vi "Save-Recall Instrument Settings.vi"(8 "error in (no error)":errorcluster, 9 "Memory Location (1)":i32(ring)=1 items=["1"=1, "2"=2, "3"=3, "4"=4], 10 "Operation (0: Save)":u16(ring) items=["Save", "Recall"], 11 "VISA resource name":refnum<visa-resource-name>) -> (0 "error out":errorcluster, 3 "VISA resource name out":refnum<visa-resource-name>)   [LabVIEW 2020, in "Agilent 34401.lvlib"]
doc: "Allows users to save or recall instrument mode at a specific memory location.\n\n<B>Note:</B>\n\n(1) This VI only applies to the 34410/34411 models.\n\n(2) Low-level <B>Initiate Measurement</B> and <B>Fetch Measurement</B> VIs must be used to transfer data from the instrument after a Recall operation. Higher level VIs like Read, configure instrument parameters that can differ from those recalled with this VI."
uses:
  Agilent 34401.lvlib
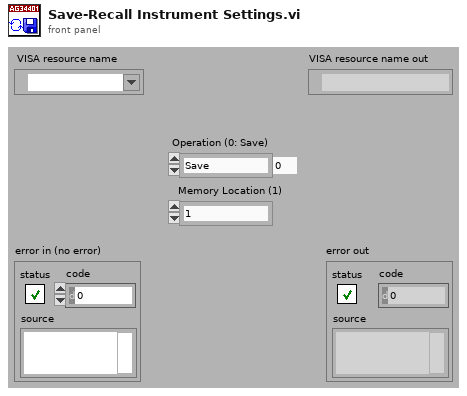
[diagram p1: front panel]
types:
  T1 = typedef "Agilent 34401.lvlib/Extended User Data.ctl" = cluster{"Trigger Source":u16, "Math Storage":u16, "Agilent Model":i32}
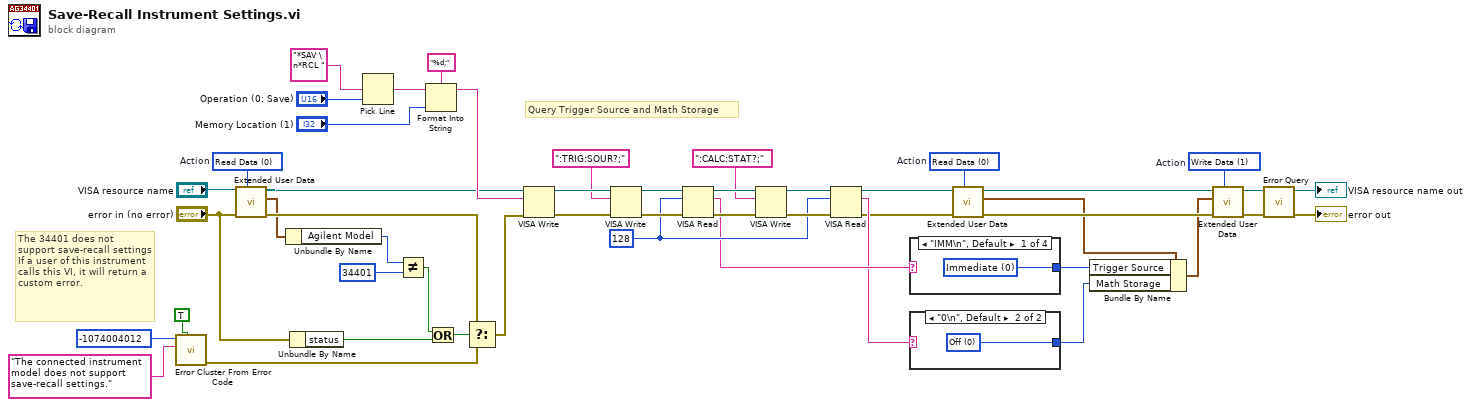
[diagram p0: block diagram]
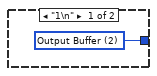
[diagram p2: hidden frame]
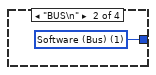
[diagram p3: hidden frame]
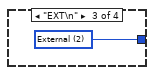
[diagram p4: hidden frame]
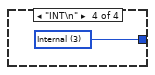
[diagram p5: hidden frame]
diagram:
  w14 = u16 0 items=["Read Data", "Write Data", "Dispose of Data"]  # Action
  w21 = u16 1 items=["Read Data", "Write Data", "Dispose of Data"]  # Action
  w6 = u32 128 ("byte count")
  w27 = u16 0 items=["Read Data", "Write Data", "Dispose of Data"]  # Action
  # "Query Trigger Source and Math Storage"
  # "The 34401 does not support save-recall settings If a user of this instrument calls this VI, it will return a custom error."
  n1 = call <vilib>:"Error Cluster From Error Code.vi"("show call chain? (False)"=TRUE, "error message (\"\")"="The connected instrument model does not support save-recall settings." ("Source (VI Name)"), "error code (0)"=-1074004012 ("Code")) -> ("error out"=w38:errorcluster)  [unwired: 6 in]
  n2 = call "Extended User Data.vi"("Action (0: Read Data)"=w27, "Error In (no error)"="error in (no error)", "VISA resource name in"="VISA resource name") -> ("Error Out"=w30:errorcluster, "User Data Out"=w20:T1, "VISA resource name out"=w29:refnum<visa-resource-name>)  [unwired: 6 in]
  n3 = Unbundle By Name(w20) -> ("Agilent Model"=w28:i32)
  n4 = Unbundle By Name("error in (no error)") -> ("status"=w34:bool)
  n5 = Pick Line(multi-line string="*SAV \n*RCL ", line index="Operation (0: Save)") -> (output string=w43:string)  [unwired: 1 in]
  n6 = Not Equal?(x=w28, y=u32 34401 ("x")) -> (x != y?=w35:bool)
  n7 = Format Into String(format string="%d;", initial string=w43, "Memory Location (1)") -> (resulting string=w45:string)  [unwired: 1 in, 1 out]
  n8 = Or(x=w35, y=w34) -> (x .or. y?=w33:bool)
  n9 = Select(t=w30, s=w33, f=w38) -> (s? t:f=w37:errorcluster)
  n10 = VISA Write(VISA resource name=w29, write buffer=w45, error in (no error)=w37) -> (VISA resource name out=w26:refnum<visa-resource-name>, error out=w25:errorcluster)  [unwired: 1 out]
  n11 = VISA Write(VISA resource name=w26, write buffer=":TRIG:SOUR?;", error in (no error)=w25) -> (VISA resource name out=w22:refnum<visa-resource-name>, error out=w23:errorcluster)  [unwired: 1 out]
  n12 = VISA Read(VISA resource name=w22, byte count=w6, error in (no error)=w23) -> (VISA resource name out=w9:refnum<visa-resource-name>, read buffer=w5:string, error out=w10:errorcluster)  [unwired: 1 out]
  n13 = VISA Write(VISA resource name=w9, write buffer=":CALC:STAT?;", error in (no error)=w10) -> (VISA resource name out=w7:refnum<visa-resource-name>, error out=w8:errorcluster)  [unwired: 1 out]
  n14 = VISA Read(VISA resource name=w7, byte count=w6, error in (no error)=w8) -> (VISA resource name out=w2:refnum<visa-resource-name>, read buffer=w4:string, error out=w3:errorcluster)  [unwired: 1 out]
  n15 = case shown="\"IMM\\n\", Default" w5 {
    tunnel: [w50 w51 w52 w53] -> w17
    frame "IMM\n", Default {
      w50 = u16 0 items=["Immediate", "Software (Bus)", "External", "Internal"] ("Trigger Source")
    }
    frame "BUS\n" {
      w51 = u16 1 items=["Immediate", "Software (Bus)", "External", "Internal"] ("Trigger Source")
    }
    frame "EXT\n" {
      w52 = u16 2 items=["Immediate", "Software (Bus)", "External", "Internal"] ("Trigger Source")
    }
    frame "INT\n" {
      w53 = u16 3 items=["Immediate", "Software (Bus)", "External", "Internal"] ("Trigger Source")
    }
  }
  n16 = case shown="\"0\\n\", Default" w4 {
    tunnel: [w54 w55] -> w16
    frame "1\n" {
      w54 = u16 2 items=["Off", "Internal Buffer", "Output Buffer"] ("Math Storage")
    }
    frame "0\n", Default {
      w55 = u16 0 items=["Off", "Internal Buffer", "Output Buffer"] ("Math Storage")
    }
  }
  n17 = call "Extended User Data.vi"("Action (0: Read Data)"=w14, "Error In (no error)"=w3, "VISA resource name in"=w2) -> ("Error Out"=w19:errorcluster, "User Data Out"=w15:T1, "VISA resource name out"=w18:refnum<visa-resource-name>)  [unwired: 6 in]
  n18 = Bundle By Name(cluster=w15, "Trigger Source"=w17, "Math Storage"=w16) -> (w13:T1)
  n19 = call "Extended User Data.vi"("Action (0: Read Data)"=w21, "Error In (no error)"=w19, "User Data In"=w13, "VISA resource name in"=w18) -> ("Error Out"=w12:errorcluster, "VISA resource name out"=w11:refnum<visa-resource-name>)  [unwired: 5 in, 1 out]
  n20 = call "Error Query.vi"("error in (no error)"=w12, "VISA resource name"=w11) -> ("error out"=→"error out":errorcluster, "VISA resource name out"=→"VISA resource name out":refnum<visa-resource-name>)  [unwired: 6 in, 2 out]
